vi "StopAndWait_SubVi.vi"(8 "error in (no error)":errorcluster, 11 "VISA Refnum in":refnum<visa-resource-name>) -> (0 "error out":errorcluster, 3 "VISA Refnum out":refnum<visa-resource-name>)   [LabVIEW 2011]
uses:
  <instrlib>/Newport ESP301/Newport ESP301.lvlib
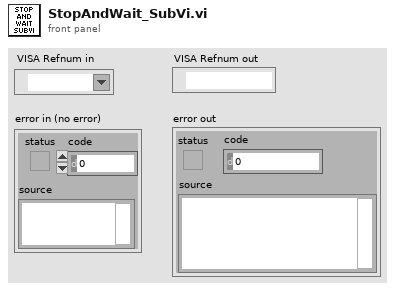
[diagram p1: front panel]
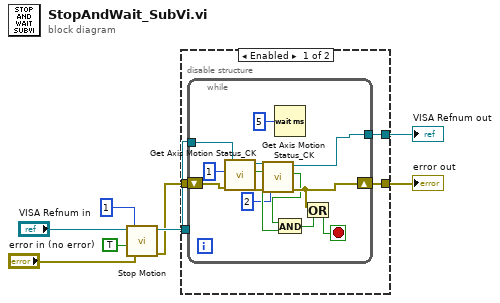
[diagram p0: block diagram]
diagram:
  n1 = call <instrlib>:"Stop Motion.vi"("error in (no error)"="error in (no error)", "Stop all axes (F)"=TRUE, "Axis (1)"=1, "VISA resource name"="VISA Refnum in") -> ("error out"=w1:errorcluster, "VISA resource name out"=w3:refnum<visa-resource-name>)  [unwired: 2 in]
  n2 = disable-structure shown="Enabled" {
    disable-tunnel: [w12 w27] -> w7
    disable-tunnel: [w11 w26] -> w5
    disable-tunnel: w3 -> [w10 w27]
    disable-tunnel: w1 -> [w9 w26]
    frame Enabled {
      n3 = while {
        tunnel: w10 -> [w25]
        shift-right: [w23] -> w11
        shift-left: w9 -> [w21]
        tunnel: [w15] -> w12
        stop <- w17 stop-if-true
        n4 = call "Get Axis Motion Status_CK.vi"("error in (no error)"=w21, "Axis (1)"=1, "VISA resource name"=w25) -> ("error out"=w22:errorcluster, "Motion Done"=w19:bool, "VISA resource name out"=w24:refnum<visa-resource-name>)  [unwired: 2 in]
        n5 = call "Get Axis Motion Status_CK.vi"("error in (no error)"=w22, "Axis (1)"=2, "VISA resource name"=w24) -> ("error out"=w23:errorcluster, "Motion Done"=w20:bool, "VISA resource name out"=w15:refnum<visa-resource-name>)  [unwired: 2 in]
        n6 = Wait (ms)(milliseconds to wait=u32 5) -> ()  [unwired: 1 out]
        n7 = And(x=w20, y=w19) -> (x .and. y?=w18:bool)
        n8 = Or(x=w23, y=w18) -> (x .or. y?=w17:bool)
      }
    }
    frame Disabled {
    }
  }
  "error out" <- w5
  "VISA Refnum out" <- w7
